vi "ChangeTableName.vi"(8 "error in (no error)":errorcluster caption="错误输入（无错误）", 10 "TableName":string, 11 "DataBase输入":refnum<class "DataBase.lvclass">) -> (0 "error out":errorcluster caption="错误输出", 3 "DataBase输出":refnum<class "DataBase.lvclass">)   [LabVIEW 2019, in "DataBase.lvlib" / "DataBase.lvclass"]
uses:
  DataBase.lvclass
  DataBase.lvclass/DataBase.ctl
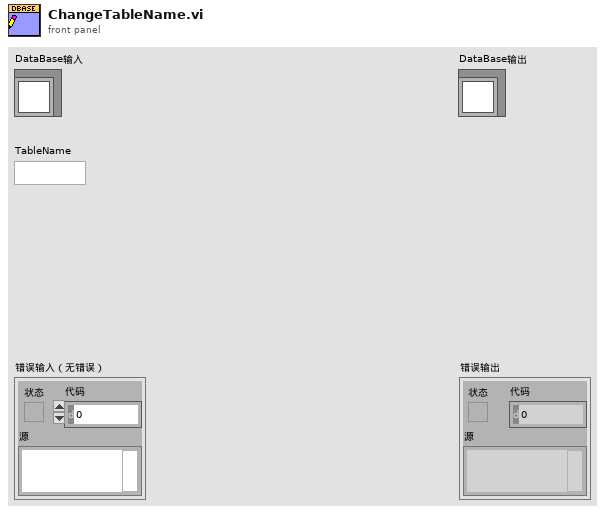
[diagram p1: front panel]
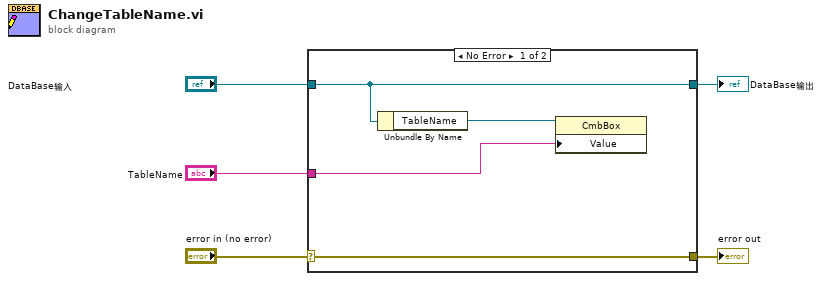
[diagram p0: block diagram]
diagram:
  n1 = case shown="No Error" "error in (no error)" {
    selector: "error in (no error)" -> [w9 w10]
    tunnel: [w9 w10] -> w4
    tunnel: [w8 w11] -> w2
    tunnel: "DataBase输入" -> [w8 w11]
    tunnel: "TableName" -> [w6 _]
    frame No Error {
      n2 = Unbundle By Name(w8) -> ("TableName"=w7:refnum<vi>)
      n3 = property class="CmbBox"(reference=w7, "Value"=w6) -> ()  [unwired: 1 in, 2 out]
    }
    frame Error {
    }
  }
  "error out" <- w4
  "DataBase输出" <- w2
